vi "Test INI Settings.vi"(11 "Test Case In":refnum<class "INI Settings.lvclass">) -> (0 "error out":errorcluster, 3 "Test Case Out":refnum<class "INI Settings.lvclass">)   [LabVIEW 2020, in "INI Settings.lvclass"]
uses:
  INI Settings.lvclass
  INI Settings.lvclass/INI Settings.ctl
  resource/plugins/lv_icon.lvlib
panel:
  in  "Font ComboBox":string(combo)
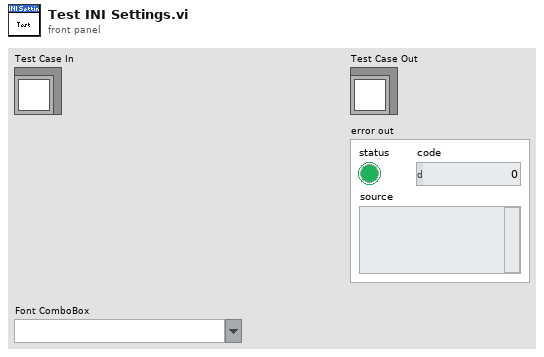
[diagram p1: front panel]
types:
  T1 = typedef "lv_icon.lvlib/INI Data.ctl" = cluster{"Show Terminals?":bool, "Text":cluster{"Font":T2, "Alignment":T3, "Size":T4}, "3rd party Templates":cluster{"Store 3rd party Templates?":bool, "Folder Name":string}, "Merge user layers on commit":bool, "Body Text":T5, "Fill Color":T6, "Edge Color":T6, "Tab":u16, "Tool":T7, "Disable Layers?":bool}
  T2 = typedef "Font.ctl" = string
  T3 = typedef "Alignment.ctl" = u16
  T4 = typedef "Font Size.ctl" = u8
  T5 = typedef "BodyText.ctl" = cluster{"Line 1 text":string, "Line 2 text":string, "Line 3 text":string, "Line 4 text":string, "Line 1 color":u32, "Line 2 color":u32, "Line 3 color":u32, "Line 4 color":u32, "Body Text Spec":cluster{"Font":T2, "Alignment":T3, "Size":u8}, "Center text vertically":bool, "Capitalize Text":bool}
  T6 = typedef "IEColor.ctl" = u32
  T7 = typedef "Tools.ctl" = enum32{"Pencil", "Line", "Dropper", "Fill", "Rectangle", "Filled Rectangle", "Ellipse", "Filled Ellipse", "Eraser", "Text", "Select", "Move"}
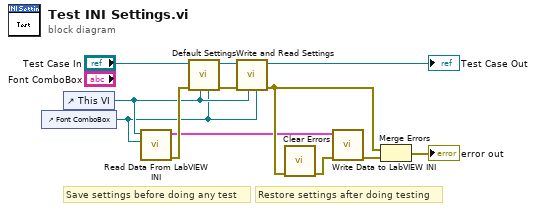
[diagram p0: block diagram]
diagram:
  # "Restore settings after doing testing"
  # "Save settings before doing any test"
  n1 = control-ref of="Font ComboBox"() -> (w2:refnum<vi>)
  n2 = control-ref of="This VI"() -> (w3:refnum<vi>)
  n3 = call "Read Data From LabVIEW INI.vi"("DNL_Font"=w2, "IE VI Ref"=w3) -> ("error out"=w12:errorcluster, "INI Data"=w5:T1)  [unwired: 8 in]
  n4 = call "Default Settings.vi"("Font ComboBox"=w2, "VI"=w3, "error in"=w12, "INI Settings in"="Test Case In") -> ("error out"=w10:errorcluster, "INI Settings out"=w4:refnum<class "INI Settings.lvclass">)  [unwired: 6 in]
  n5 = call "Write and Read Settings.vi"("Font ComboBox"=w2, "VI"=w3, "error in"=w10, "INI Settings in"=w4) -> ("error out"=w7:errorcluster, "INI Settings out"=→"Test Case Out":refnum<class "INI Settings.lvclass">)  [unwired: 6 in]
  n6 = call <vilib>:"Clear Errors.vi"("error in (no error)"=w7) -> ("error out"=w8:errorcluster)  [unwired: 5 in, 1 out]
  n7 = call "Write Data to LabVIEW INI.vi"("error in"=w8, "INI Data"=w5) -> ("error out"=w11:errorcluster)  [unwired: 9 in]
  n8 = Merge Errors(w7, w11) -> (→"error out":errorcluster)
